vi "main_controller.vi"(8 "error in":errorcluster) -> (0 "error out":errorcluster)   [LabVIEW 2020]
uses:
  #typedefs/#typedef_enum_QueueActions.ctl
  #typedefs/#typedef_cluster_CTRL_QueueData.ctl
  #typedefs/#typedef_enum_CTRL_States.ctl
  #typedefs/#typedef_cluster_ANALYZE_QueueData.ctl
  #typedefs/#typedef_enum_ANALYZE_States.ctl
  #typedefs/#typedef_cluster_GUI_QueueData.ctl
  #typedefs/#typedef_enum_GUI_States.ctl
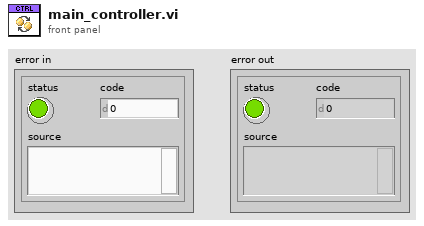
[diagram p1: front panel]
types:
  T1 = typedef "#typedef_cluster_CTRL_QueueData.ctl" = cluster{"Cmd":T2, "Variant":variant}
  T2 = typedef "#typedef_enum_CTRL_States.ctl" = enum16{"Init", "AnalyzeImage", "SaveImage", "ErrorHandling", "ExitRequest", "Exit"}
  T3 = typedef "#typedef_enum_QueueActions.ctl" = enum16{"Obtain", "GetRef", "Enqueue", "Release"}
  T4 = typedef "#typedef_enum_ANALYZE_States.ctl" = enum16{"Init", "Open", "UpdateOptions", "Process", "Save", "ErrorHandling", "ExitRequest", "Exit"}
  T5 = typedef "#typedef_cluster_ANALYZE_QueueData.ctl" = cluster{"Cmd":T4, "Variant":variant}
  T6 = typedef "#typedef_enum_GUI_States.ctl" = enum16{"Init", "AddImages", "PreviousImage", "NextImage", "AnalyzeImage", "SaveImage", "GenFakeError", "ErrorHandling", "ExitRequest", "Exit"}
  T7 = typedef "#typedef_cluster_GUI_QueueData.ctl" = cluster{"Cmd":T6, "Variant":variant}
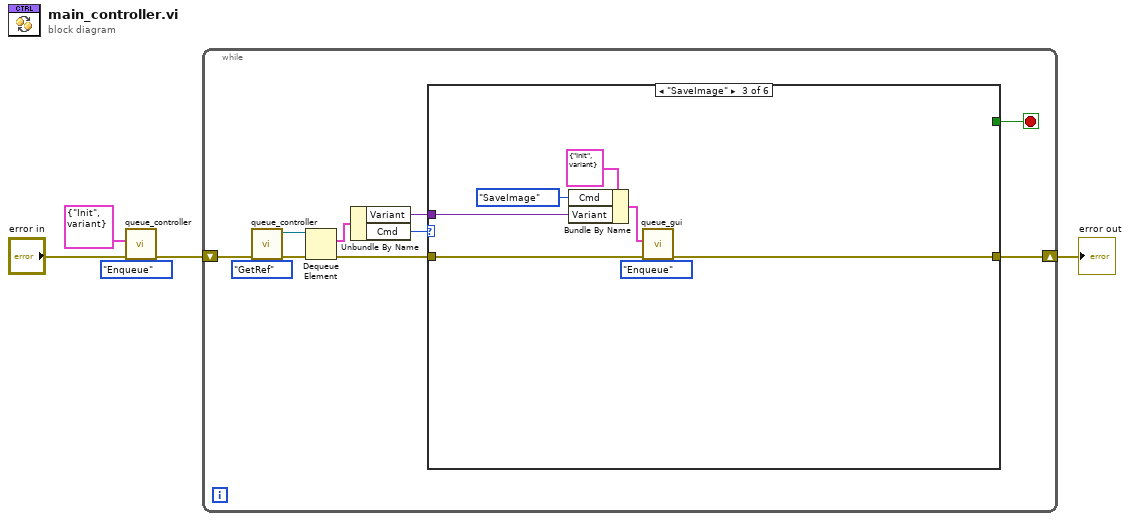
[diagram p0: block diagram]
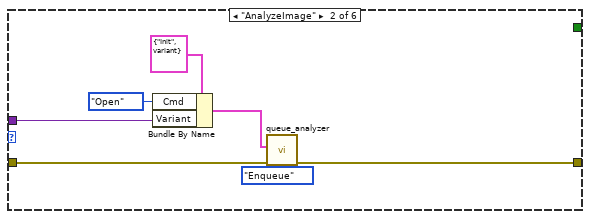
[diagram p3: hidden frame]
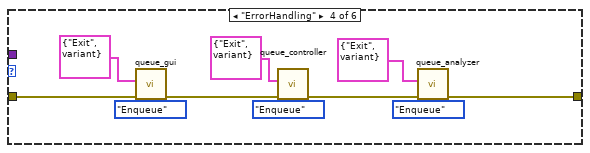
[diagram p4: hidden frame]
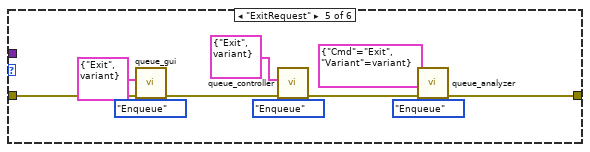
[diagram p5: hidden frame]
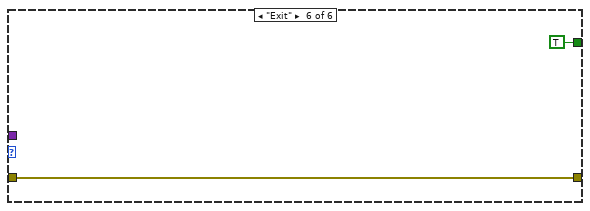
[diagram p6: hidden frame]
diagram:
  n1 = call "queue_controller.vi"("QueueActions"=#typedef_enum_QueueActions."Enqueue", "error in (no error)"="error in", "QueueDataIn"=T1 {"Cmd"=enum."Init", "Variant"=variant}) -> ("error out"=w4:errorcluster)  [unwired: 7 in, 1 out]
  n2 = while {
    shift-right: [w8] -> w5
    shift-left: w4 -> [w14]
    stop <- w7 stop-if-true
    n3 = call "queue_controller.vi"("QueueActions"=#typedef_enum_QueueActions."GetRef", "error in (no error)"=w14) -> ("error out"=w12:errorcluster, "queue out"=w13:refnum<queue>)  [unwired: 8 in]
    n4 = Dequeue Element(queue=w13, error in (no error)=w12) -> (element=w11:T1, error out=w9:errorcluster)  [unwired: 1 in, 2 out]
    n5 = Unbundle By Name(w11) -> ("Variant"=w6:variant, "Cmd"=w10:T2)
    n6 = case shown="\"SaveImage\"" w10 {
      tunnel: w9 -> [w16 w23 w26 w40 w50 w52]
      tunnel: [w16 w22 w30 w33 w43 w52] -> w8
      tunnel: [_ _ _ _ _ TRUE] -> w7
      tunnel: w6 -> [_ w20 w27 _ _ _]
      frame "Init", Default {
      }
      frame "AnalyzeImage" {
        n7 = Bundle By Name(cluster=T5 {"Cmd"=enum."Init", "Variant"=variant} ("QueueDataIn"), "Cmd"=#typedef_enum_ANALYZE_States."Open", "Variant"=w20) -> (w18:T5)
        n8 = call "queue_analyzer.vi"("QueueActions"=#typedef_enum_QueueActions."Enqueue", "error in (no error)"=w23, "QueueDataIn"=w18) -> ("error out"=w22:errorcluster)  [unwired: 7 in, 1 out]
      }
      frame "SaveImage" {
        n9 = Bundle By Name(cluster=T7 {"Cmd"=enum."Init", "Variant"=variant} ("QueueDataIn"), "Cmd"=#typedef_enum_GUI_States."SaveImage", "Variant"=w27) -> (w24:T7)
        n10 = call "queue_gui.vi"("QueueActions"=#typedef_enum_QueueActions."Enqueue", "error in (no error)"=w26, "QueueDataIn"=w24) -> ("error out"=w30:errorcluster)  [unwired: 7 in, 1 out]
      }
      frame "ErrorHandling" {
        n11 = call "queue_gui.vi"("QueueActions"=#typedef_enum_QueueActions."Enqueue", "error in (no error)"=w40, "QueueDataIn"=T7 {"Cmd"=enum."Exit", "Variant"=variant}) -> ("error out"=w39:errorcluster)  [unwired: 7 in, 1 out]
        n12 = call "queue_controller.vi"("QueueActions"=#typedef_enum_QueueActions."Enqueue", "error in (no error)"=w39, "QueueDataIn"=T1 {"Cmd"=enum."Exit", "Variant"=variant}) -> ("error out"=w34:errorcluster)  [unwired: 7 in, 1 out]
        n13 = call "queue_analyzer.vi"("QueueActions"=#typedef_enum_QueueActions."Enqueue", "error in (no error)"=w34, "QueueDataIn"=T5 {"Cmd"=enum."Exit", "Variant"=variant}) -> ("error out"=w33:errorcluster)  [unwired: 7 in, 1 out]
      }
      frame "ExitRequest" {
        n14 = call "queue_gui.vi"("QueueActions"=#typedef_enum_QueueActions."Enqueue", "error in (no error)"=w50, "QueueDataIn"=T7 {"Cmd"=enum."Exit", "Variant"=variant}) -> ("error out"=w49:errorcluster)  [unwired: 7 in, 1 out]
        n15 = call "queue_controller.vi"("QueueActions"=#typedef_enum_QueueActions."Enqueue", "error in (no error)"=w49, "QueueDataIn"=T1 {"Cmd"=enum."Exit", "Variant"=variant}) -> ("error out"=w44:errorcluster)  [unwired: 7 in, 1 out]
        n16 = call "queue_analyzer.vi"("QueueActions"=#typedef_enum_QueueActions."Enqueue", "error in (no error)"=w44, "QueueDataIn"=T5 {"Cmd"=enum."Exit", "Variant"=variant}) -> ("error out"=w43:errorcluster)  [unwired: 7 in, 1 out]
      }
      frame "Exit" {
      }
    }
  }
  "error out" <- w5
